vi "clFileReader_initReader.vi"(9 "DataLenght":u32, 10 "HiddenOffset":u32, 11 "clFile.lvclass":refnum<class "clFile.lvclass">) -> (3 "clFileReader.lvclass":refnum<class "clFileReader.lvclass">)   [LabVIEW 2020, in "vi_lib.lvlib" / "clFileReader.lvclass"]
uses:
  clFileReader.lvclass
  clFile/clFile.lvclass
  clFileReader.lvclass/clFileReader.ctl
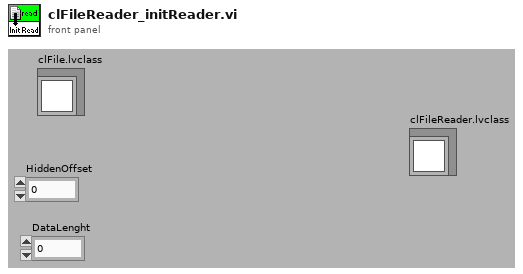
[diagram p1: front panel]
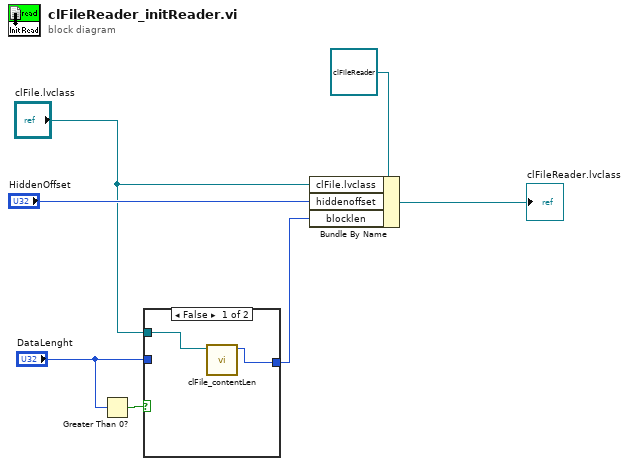
[diagram p0: block diagram]
diagram:
  n1 = Greater Than 0?(x="DataLenght") -> (x > 0?=w5:bool)
  n2 = case shown="False" w5 {
    tunnel: "DataLenght" -> [_ w10]
    tunnel: [w9 w10] -> w3
    tunnel: "clFile.lvclass" -> [w8 _]
    frame False {
      n3 = call "clFile_contentLen.vi"("clFile.lvclass"=w8) -> ("length"=w9:u32)  [unwired: 10 out]
    }
    frame True {
    }
  }
  n4 = Bundle By Name(cluster=refnum<class "clFileReader.lvclass"> refnum ("clFileReader.lvclass"), "clFile.lvclass"="clFile.lvclass", "hiddenoffset"="HiddenOffset", "blocklen"=w3) -> (→"clFileReader.lvclass":refnum<class "clFileReader.lvclass">)
